vi "Find BBox Center (SubVI).vi"(11 "BBox Array In":i32[][](array[numeric])) -> (0 "Center Array":i32[][](array[numeric]), 3 "BBox Array Out":i32[][](array[numeric]))   [LabVIEW 2020]
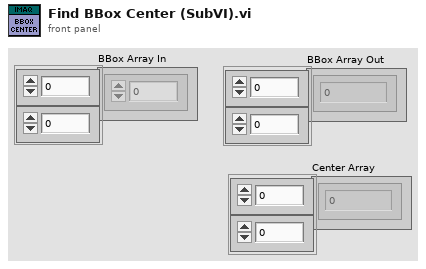
[diagram p1: front panel]
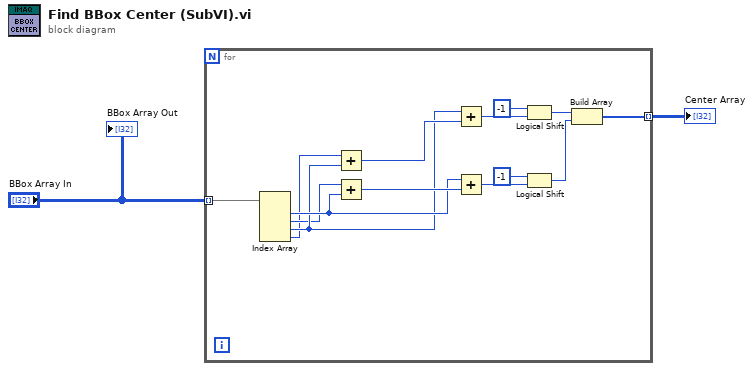
[diagram p0: block diagram]
diagram:
  n1 = for {
    tunnel: "BBox Array In" -> [w16] mode=indexing
    tunnel: [w15] -> w1 mode=indexing
    n2 = Index Array(array=w16) -> (element #1=w7:i32, element #2=w4:i32, element #3=w5:i32, element #4=w3:i32)  [unwired: 4 in]
    n3 = Add(x=w3, y=w5) -> (x+y=w6:i32)
    n4 = Add(x=w4, y=w7) -> (x+y=w8:i32)
    n5 = Add(x=w5, y=w6) -> (x+y=w9:i32)
    n6 = Add(x=w7, y=w8) -> (x+y=w12:i32)
    n7 = Logical Shift(y=i16 -1, x=w9) -> (x << y=w13:i32)
    n8 = Logical Shift(y=i16 -1, x=w12) -> (x << y=w14:i32)
    n9 = Build Array(w13, w14) -> (w15:i32[])
  }
  "Center Array" <- w1
  "BBox Array Out" <- "BBox Array In"
